vi "X360 Button Get Value.vi"(6 "Player":bool=TRUE, 9 "Button":T2(ring), 10 "Joystick 2 values":T1, 11 "Joystick 1 values":T1) -> (0 "Button pressed":bool=TRUE, 1 "Double output":dbl format="%#_13g", 2 "Joystick 2 values Out":T1, 3 "Joystick 1 values Out":T1)   [LabVIEW 2015]
panel:
  in  "Input Deadband":dbl=0.1 min=0.0 max=1.0 step=0.1
  in  "Deadband Upper Limit":dbl=1.0 min=0.0 max=1.0 step=0.1 format="%#_13g"
  in  "Use Deadband":bool=TRUE
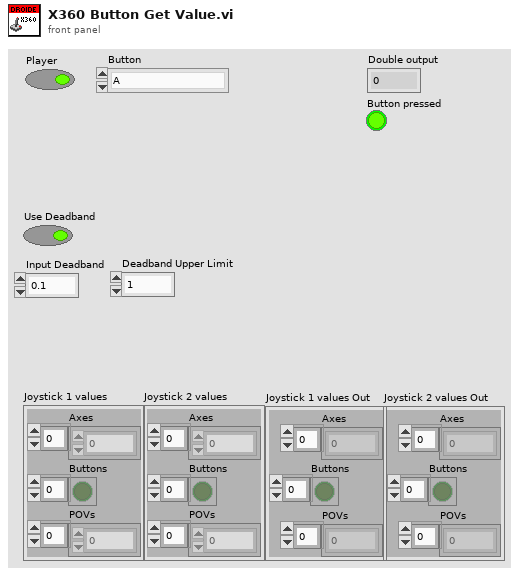
[diagram p1: front panel]
types:
  T1 = cluster{"Axes":dbl[], "Buttons":bool[], "POVs":i16[]}
  T2 = enum16{"A", "B", "X", "Y", "LB", "RB", "Select", "Start", "StickClick Left", "StickClick Right", "Stick Left X", "Stick Left Y", "Left Trigger", "Right Trigger", "Stick Right X", "Stick Right Y"}
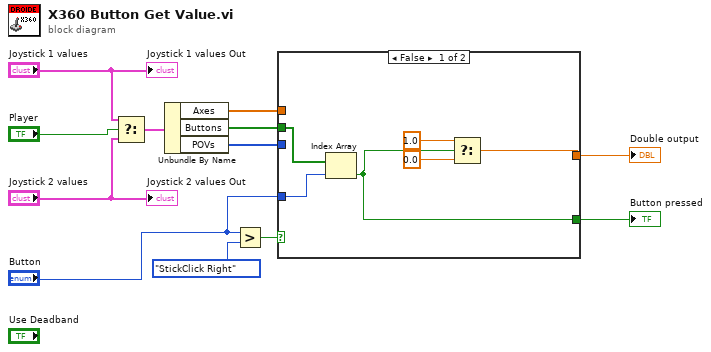
[diagram p0: block diagram]
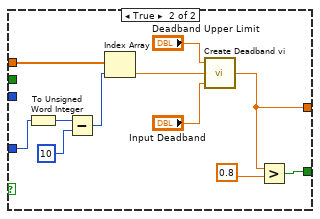
[diagram p2: hidden frame]
diagram:
  n1 = Select(t="Joystick 1 values", s="Player", f="Joystick 2 values") -> (s? t:f=w7:T1)
  n2 = Unbundle By Name(w7) -> ("Axes"=w6:dbl[], "Buttons"=w5:bool[], "POVs"=w4:i16[])
  n3 = Greater?(x="Button", y=T2."StickClick Right") -> (0:w10:bool)
  n4 = case shown="False" w10 {
    tunnel: "Button" -> [w18 w29]
    tunnel: [w16 w21] -> w9
    tunnel: [w13 w27] -> w8
    tunnel: w6 -> [_ w25]
    tunnel: w5 -> [w17 _]
    tunnel: w4 -> [_ _]
    frame False {
      n5 = Index Array(array=w17, index=w18) -> (element=w13:bool)
      n6 = Select(t=1.0, s=w13, f=0.0) -> (s? t:f=w16:dbl)
    }
    frame True {
      n7 = To Unsigned Word Integer(number=w29) -> (unsigned 16bit integer=w24:u16)
      n8 = Subtract(x=w24, y=u16 10) -> (x-y=w22:u16)
      n9 = Index Array(array=w25, index=w22) -> (element=w26:dbl)
      n10 = call "Create Deadband vi.vi"("Input Deadband"="Input Deadband", "Input"=w26, "Output Upper Limit"="Deadband Upper Limit") -> ("Output"=w21:dbl)  [unwired: 1 in]
      n11 = Greater?(x=w21, y=0.8) -> (0:w27:bool)
    }
  }
  "Double output" <- w9
  "Button pressed" <- w8
  "Joystick 1 values Out" <- "Joystick 1 values"
  "Joystick 2 values Out" <- "Joystick 2 values"
